vi "Set_Gen_ConfL0SUM.vi"(0 "AWG VISA":refnum<visa-resource-name>="AgilentGenerator1", 5 "error in (no error)":errorcluster) -> (12 "Amplitude 1 OUT":dbl=0.5, 13 "Amplitude 2 OUT":dbl=1.0, 14 "VISA resource name out":refnum<visa-resource-name>="AgilentGenerator1", 15 "Pulse Width in seconds 1 OUT":dbl=3e-09, 16 "Trigger Level 1":dbl=0.025, 17 "Trigger Level 2":dbl, 18 "Pulse Width in seconds 2 OUT":dbl=2e-08, 19 "error out":errorcluster)   [LabVIEW 2012]
uses:
  C/Program Files/National Instruments/LabVIEW 2012/instr.lib/Agilent 81150/Agilent 81150.lvlib
panel:
  in  "Delay 2 ( Seconds)":dbl
  in  "Delay 1 (Seconds)":dbl
  in  "Pulse Width in seconds 2":dbl=2e-08
  in  "Frequency 2":dbl=10000000.0
  in  "Amplitude 2":dbl=1.0
  in  "Pulse Width in seconds 1":dbl=3e-09
  in  "Frequency 1":dbl=12000000.0
  in  "Amplitude 1":dbl=0.5
  in  "Trigger Mode 2":u16(ring) items=["Edge", "Level"]
  in  "Trigger Source 2":u16(ring)=1 items=["Immediate", "Internal", "External", "Software Trigger Function"]
  in  "Channel 2":u16(ring)=2 items=["Channel1"=1, "Channel2"=2]
  in  "Enable Burst 2":bool
  in  "Trigger Slope 2":u16(ring) items=["Positive", "Negative", "Either"]
  in  "Burst Count 2":i32=10000
  in  "TriggerFrequency 2":dbl=100000.0
  in  "DC Offset 2":dbl
  in  "Waveform  2":u16(ring)=4 items=["Sine", "Square", "Ramp Up", "Ramp Down", "Pulse", "Noise", "DC"]
  in  "Leading Edge Time  2":dbl=1e-09
  in  "Trailing Edge Time  2":dbl=1e-09
  in  "Trailing Edge Time 1":dbl=1.5e-09
  in  "Leading Edge Time 1":dbl=1.5e-09
  in  "Waveform 1":u16(ring)=4 items=["Sine", "Square", "Ramp Up", "Ramp Down", "Pulse", "Noise", "DC"]
  in  "DC Offset 1":dbl
  in  "Trigger Frequency 1":dbl=10000.0
  in  "Burst Count 1":i32=1000
  in  "Trigger Slope 1":u16(ring) items=["Positive", "Negative", "Either"]
  in  "Enable Burst":bool
  in  "Channel 1":u16(ring)=1 items=["Channel1"=1, "Channel2"=2]
  in  "Trigger Source 1":u16(ring)=1 items=["Immediate", "Internal", "External", "Software Trigger Function"]
  in  "Trigger Mode 1":u16(ring) items=["Edge", "Level"]
  in  "Channel 2":bool
  in  "Channel 1":bool=TRUE
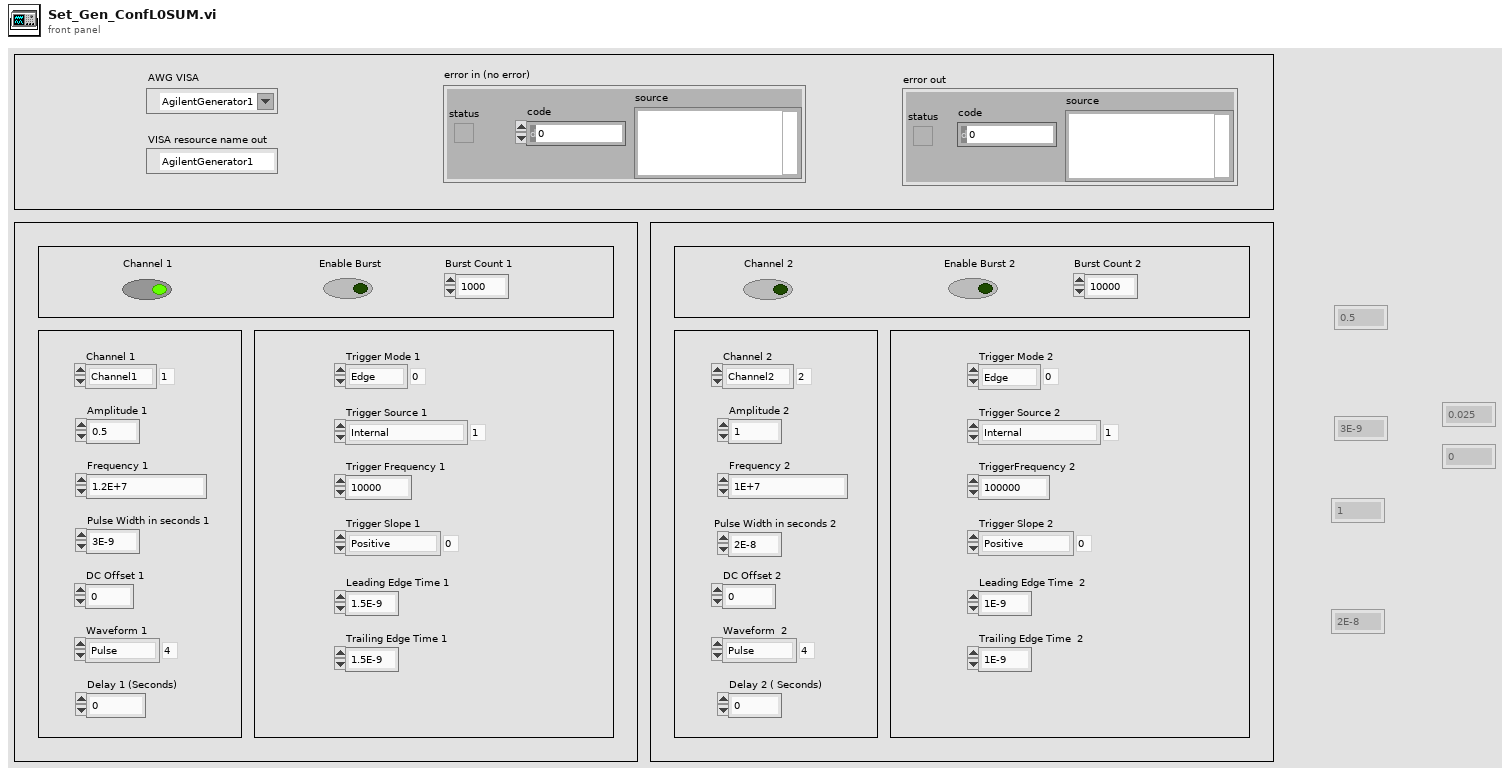
[diagram p1: front panel]
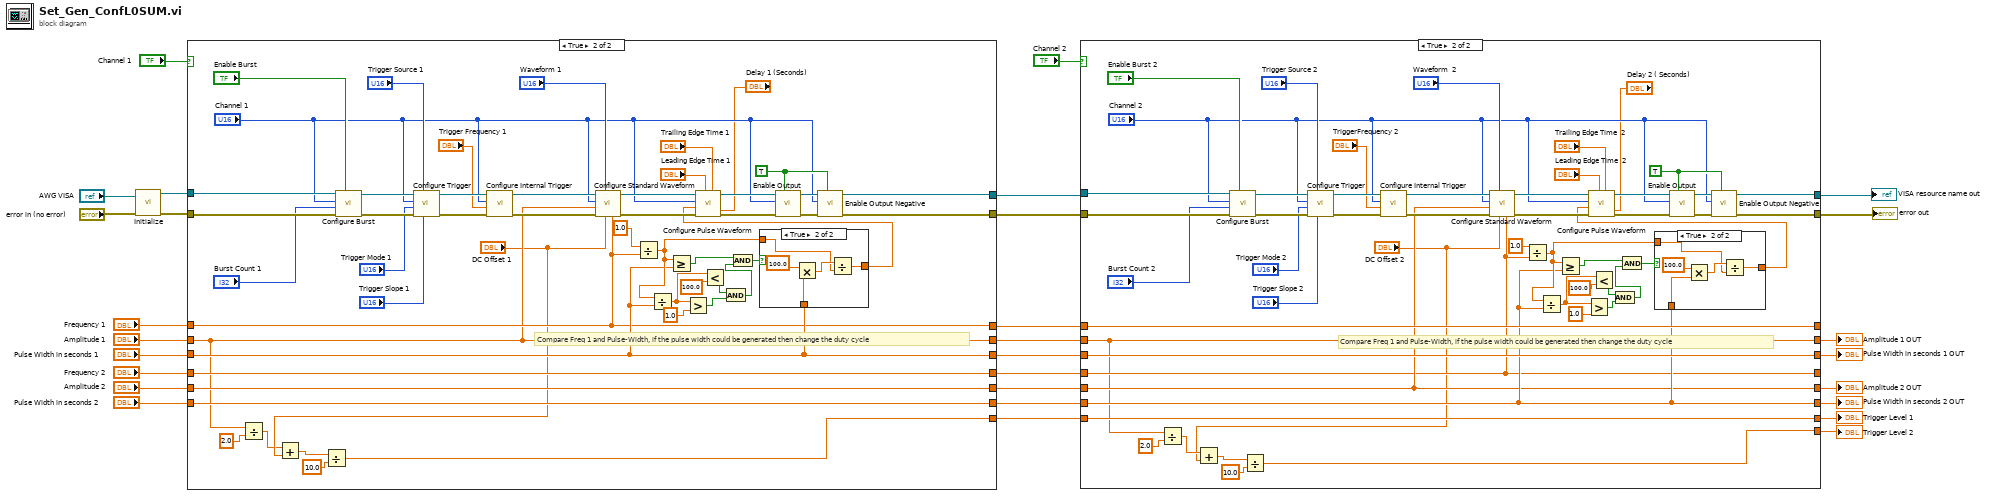
[diagram p0: block diagram]
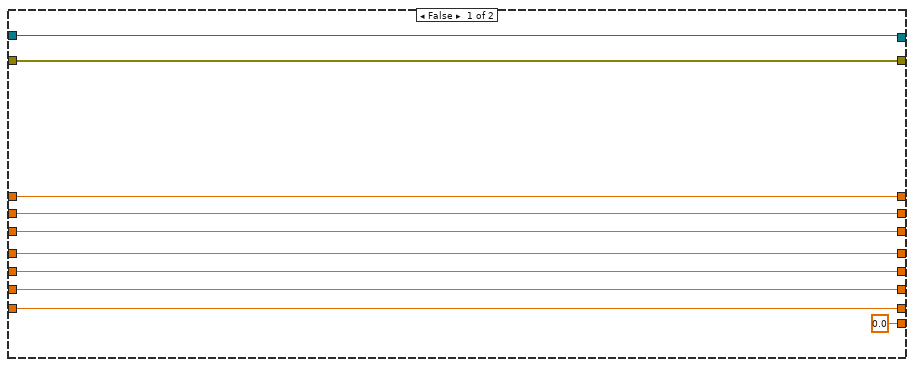
[diagram p2: hidden frame]
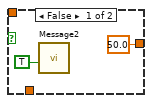
[diagram p3: hidden frame]
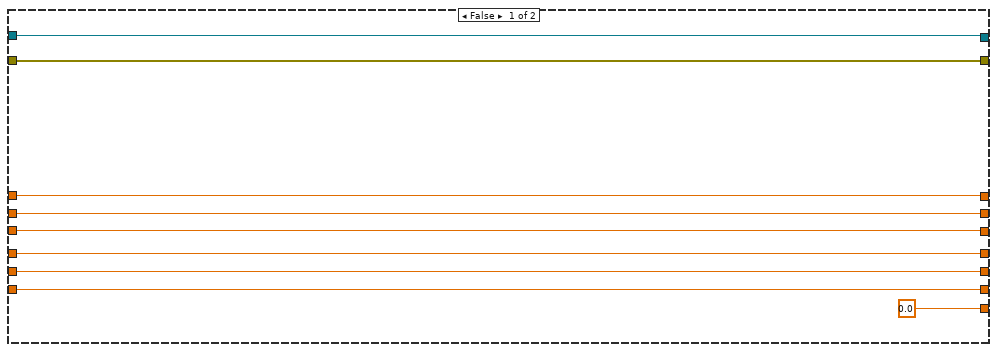
[diagram p4: hidden frame]
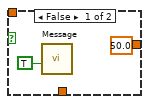
[diagram p5: hidden frame]
diagram:
  n1 = call <instrlib>:"Initialize.vi"("error in (no error)"="error in (no error)", "VISA resource name"="AWG VISA") -> ("error out"=w25:errorcluster, "VISA resource name out"=w26:refnum<visa-resource-name>)  [unwired: 8 in]
  n2 = case shown="True" "Channel 1" {
    tunnel: w26 -> [w38 w89]
    tunnel: w25 -> [w37 w88]
    tunnel: [w38 w63] -> w23
    tunnel: [w37 w62] -> w22
    tunnel: [w34 w52] -> w19
    tunnel: "Pulse Width in seconds 1" -> [w34 w52]
    tunnel: "Amplitude 1" -> [w35 w45]
    tunnel: "Frequency 1" -> [w36 w51]
    tunnel: [w36 w51] -> w14
    tunnel: [w35 w45] -> w15
    tunnel: "Frequency 2" -> [w33 w49]
    tunnel: "Amplitude 2" -> [w32 w48]
    tunnel: "Pulse Width in seconds 2" -> [w31 w47]
    tunnel: [w33 w49] -> w10
    tunnel: [w32 w48] -> w9
    tunnel: [w31 w47] -> w8
    tunnel: [0.0 w39] -> w3
    frame False {
    }
    frame True {
      w69 = TRUE ("Enable Output (T: Enable)")
      # "Compare Freq 1 and Pulse-Width, if the pulse width could be generated then change the duty cycle"
      n3 = Divide(x=w45, y=2.0) -> (x/y=w43:dbl)
      n4 = Add(x=w43, y="DC Offset 1") -> (x+y=w41:dbl)
      n5 = Divide(x=w41, y=10.0) -> (x/y=w39:dbl)
      n6 = call <instrlib>:"Configure Burst.vi"("Enable Burst (F: Disable)"="Enable Burst", "error in (no error)"=w88, "Burst Count (2)"="Burst Count 1", "Channel (1: Channel1)"="Channel 1", "VISA resource name"=w89) -> ("error out"=w86:errorcluster, "VISA resource name out"=w87:refnum<visa-resource-name>)  [unwired: 5 in]
      n7 = call <instrlib>:"Configure Trigger.vi"("Trigger Slope (0: Positive)"="Trigger Slope 1", "Trigger Source (0: Immediate)"="Trigger Source 1", "error in (no error)"=w86, "Trigger Mode (0: Edge)"="Trigger Mode 1", "Channel (1: Channel1)"="Channel 1", "VISA resource name"=w87) -> ("error out"=w79:errorcluster, "VISA resource name out"=w80:refnum<visa-resource-name>)  [unwired: 4 in]
      n8 = call "Configure Internal Trigger.vi"("error in (no error)"=w79, "Frequency (100000.0 Hz)"="Trigger Frequency 1", "Channel (1: Channel1)"="Channel 1", "VISA resource name"=w80) -> ("error out"=w77:errorcluster, "VISA resource name out"=w78:refnum<visa-resource-name>)  [unwired: 6 in]
      n9 = call <instrlib>:"Configure Standard Waveform.vi"("Frequency (1000.0 Hz)"=w51, "DC Offset (0.0 Volts)"="DC Offset 1", "Waveform (0: Sine)"="Waveform 1", "error in (no error)"=w77, "Amplitude (1.0 Vpp)"=w45, "Channel (1: Channel1)"="Channel 1", "VISA resource name"=w78) -> ("error out"=w74:errorcluster, "VISA resource name out"=w75:refnum<visa-resource-name>)  [unwired: 3 in]
      n10 = Divide(x=1.0 ("y"), y=w51) -> (x/y=w59:dbl)
      n11 = Divide(x=w59, y=w52) -> (x/y=w57:dbl)
      n12 = Greater Or Equal?(x=w59, y=w52) -> (x >= y?=w60:bool)
      n13 = Greater?(x=w57, y=1.0) -> (0:w54:bool)
      n14 = Less?(x=w57, y=100.0) -> (x < y?=w55:bool)
      n15 = And(x=w55, y=w54) -> (x .and. y?=w53:bool)
      n16 = And(x=w60, y=w53) -> (x .and. y?=w61:bool)
      n17 = case shown="True" w61 {
        tunnel: w52 -> [_ w96]
        tunnel: w59 -> [_ w92]
        tunnel: [50.0 w94] -> w50
        frame False {
          n18 = call "Message"("Enable"=TRUE) -> ()  [unwired: 9 in, 2 out]
        }
        frame True {
          n19 = Multiply(x=100.0, y=w96) -> (x*y=w93:dbl)
          n20 = Divide(x=w93, y=w92) -> (x/y=w94:dbl)
        }
      }
      n21 = call <instrlib>:"Configure Pulse Waveform.vi"("Trailing Edge Time (7.5E-9 Seconds)"="Trailing Edge Time 1", "Delay (0.0 Seconds)"="Delay 1 (Seconds)", "Leading Edge Time (7.5E-9 Seconds)"="Leading Edge Time 1", "error in (no error)"=w74, "Duty Cycle (50.0 %)"=w50, "Channel (1: Channel1)"="Channel 1", "VISA resource name"=w75) -> ("error out"=w72:errorcluster, "VISA resource name out"=w73:refnum<visa-resource-name>)  [unwired: 3 in]
      n22 = call <instrlib>:"Enable Output.vi"("Enable Output (T: Enable)"=w69, "error in (no error)"=w72, "Channel (1: Channel1)"="Channel 1", "VISA resource name"=w73) -> ("error out"=w70:errorcluster, "VISA resource name out"=w71:refnum<visa-resource-name>)  [unwired: 6 in]
      n23 = call "Enable Output Negative.vi"("Enable Output (T: Enable)"=w69, "error in (no error)"=w70, "Channel (1: Channel1)"="Channel 1", "VISA resource name"=w71) -> ("error out"=w62:errorcluster, "VISA resource name out"=w63:refnum<visa-resource-name>)  [unwired: 6 in]
    }
  }
  n24 = case shown="True" "Channel 2" {
    tunnel: w23 -> [w106 w158]
    tunnel: w22 -> [w105 w157]
    tunnel: [w106 w132] -> w21
    tunnel: [w105 w131] -> w20
    tunnel: w19 -> [w102 w119]
    tunnel: w15 -> [w103 w109]
    tunnel: w14 -> [w104 w120]
    tunnel: w10 -> [w101 w116]
    tunnel: w9 -> [w100 w117]
    tunnel: w8 -> [w99 w118]
    tunnel: [w104 w120] -> _
    tunnel: [w103 w109] -> w6
    tunnel: [w102 w119] -> w5
    tunnel: [w101 w116] -> _
    tunnel: [w100 w117] -> w4
    tunnel: [w99 w118] -> w7
    tunnel: w3 -> [w98 w114]
    tunnel: [w98 w114] -> w2
    tunnel: [0.0 w107] -> w1
    frame False {
    }
    frame True {
      w138 = TRUE ("Enable Output (T: Enable)")
      # "Compare Freq 1 and Pulse-Width, if the pulse width could be generated then change the duty cycle"
      n25 = Divide(x=w109, y=2.0) -> (x/y=w110:dbl)
      n26 = Add(x=w110, y="DC Offset 2") -> (x+y=w112:dbl)
      n27 = call <instrlib>:"Configure Burst.vi"("Enable Burst (F: Disable)"="Enable Burst 2", "error in (no error)"=w157, "Burst Count (2)"="Burst Count 2", "Channel (1: Channel1)"="Channel 2", "VISA resource name"=w158) -> ("error out"=w155:errorcluster, "VISA resource name out"=w156:refnum<visa-resource-name>)  [unwired: 5 in]
      n28 = Divide(x=w112, y=10.0) -> (x/y=w107:dbl)
      n29 = call <instrlib>:"Configure Trigger.vi"("Trigger Slope (0: Positive)"="Trigger Slope 2", "Trigger Source (0: Immediate)"="Trigger Source 2", "error in (no error)"=w155, "Trigger Mode (0: Edge)"="Trigger Mode 2", "Channel (1: Channel1)"="Channel 2", "VISA resource name"=w156) -> ("error out"=w148:errorcluster, "VISA resource name out"=w149:refnum<visa-resource-name>)  [unwired: 4 in]
      n30 = call "Configure Internal Trigger.vi"("error in (no error)"=w148, "Frequency (100000.0 Hz)"="TriggerFrequency 2", "Channel (1: Channel1)"="Channel 2", "VISA resource name"=w149) -> ("error out"=w146:errorcluster, "VISA resource name out"=w147:refnum<visa-resource-name>)  [unwired: 6 in]
      n31 = call <instrlib>:"Configure Standard Waveform.vi"("Frequency (1000.0 Hz)"=w116, "DC Offset (0.0 Volts)"="DC Offset 2", "Waveform (0: Sine)"="Waveform  2", "error in (no error)"=w146, "Amplitude (1.0 Vpp)"=w117, "Channel (1: Channel1)"="Channel 2", "VISA resource name"=w147) -> ("error out"=w143:errorcluster, "VISA resource name out"=w144:refnum<visa-resource-name>)  [unwired: 3 in]
      n32 = Divide(x=1.0 ("y"), y=w116) -> (x/y=w123:dbl)
      n33 = Divide(x=w123, y=w118) -> (x/y=w128:dbl)
      n34 = Greater Or Equal?(x=w123, y=w118) -> (x >= y?=w130:bool)
      n35 = Greater?(x=w128, y=1.0) -> (0:w125:bool)
      n36 = Less?(x=w128, y=100.0) -> (x < y?=w126:bool)
      n37 = And(x=w126, y=w125) -> (x .and. y?=w121:bool)
      n38 = And(x=w130, y=w121) -> (x .and. y?=w122:bool)
      n39 = case shown="True" w122 {
        tunnel: w118 -> [_ w162]
        tunnel: w123 -> [_ w161]
        tunnel: [50.0 w164] -> w133
        frame False {
          n40 = call "Message2"("Enable"=TRUE) -> ()  [unwired: 9 in, 2 out]
        }
        frame True {
          n41 = Multiply(x=100.0, y=w162) -> (x*y=w163:dbl)
          n42 = Divide(x=w163, y=w161) -> (x/y=w164:dbl)
        }
      }
      n43 = call <instrlib>:"Configure Pulse Waveform.vi"("Trailing Edge Time (7.5E-9 Seconds)"="Trailing Edge Time  2", "Delay (0.0 Seconds)"="Delay 2 ( Seconds)", "Leading Edge Time (7.5E-9 Seconds)"="Leading Edge Time  2", "error in (no error)"=w143, "Duty Cycle (50.0 %)"=w133, "Channel (1: Channel1)"="Channel 2", "VISA resource name"=w144) -> ("error out"=w141:errorcluster, "VISA resource name out"=w142:refnum<visa-resource-name>)  [unwired: 3 in]
      n44 = call <instrlib>:"Enable Output.vi"("Enable Output (T: Enable)"=w138, "error in (no error)"=w141, "Channel (1: Channel1)"="Channel 2", "VISA resource name"=w142) -> ("error out"=w139:errorcluster, "VISA resource name out"=w140:refnum<visa-resource-name>)  [unwired: 6 in]
      n45 = call "Enable Output Negative.vi"("Enable Output (T: Enable)"=w138, "error in (no error)"=w139, "Channel (1: Channel1)"="Channel 2", "VISA resource name"=w140) -> ("error out"=w131:errorcluster, "VISA resource name out"=w132:refnum<visa-resource-name>)  [unwired: 6 in]
    }
  }
  "VISA resource name out" <- w21
  "error out" <- w20
  "Amplitude 1 OUT" <- w6
  "Pulse Width in seconds 1 OUT" <- w5
  "Amplitude 2 OUT" <- w4
  "Pulse Width in seconds 2 OUT" <- w7
  "Trigger Level 1" <- w2
  "Trigger Level 2" <- w1
